vi "getPositionWithTime_32Bit.vi"(0 "connection ID":refnum<k5>, 1 "axis":i32, 5 "error":errorcluster) -> (14 "connection ID out":refnum<k5>, 15 "axis_out":i32, 16 "Monotonic_time_sec":i32, 17 "Monotonic_time_nsec":i32, 18 "position":dbl, 19 "error out":errorcluster)   [LabVIEW 2016, in "amc_api.lvlib"]
doc: "This function gets the current position of the positioner and provides time-information to the position."
uses:
  amc_api.lvlib
panel:
  out "jsonRespIn":string
  out "JSON-response":string="{\"jsonrpc\":\"2.0\",\"method\":\"\",\"params\":[5,1.245,true,\"name\"],\"id\":\"1\"}"
  out "JSON request":string
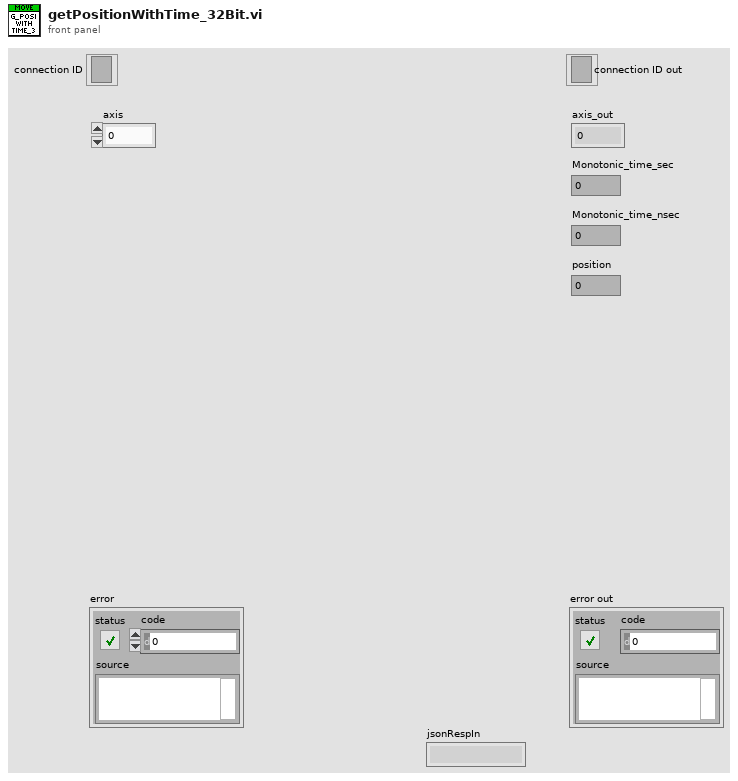
[diagram p1: front panel]
types:
  T1 = cluster{"jsonrpc":string, "method":string, "params":string[], "id":string, "api":i32, "pid":string}
  T2 = enum16{"Standard", "Buffered", "CRLF", "Immediate"}
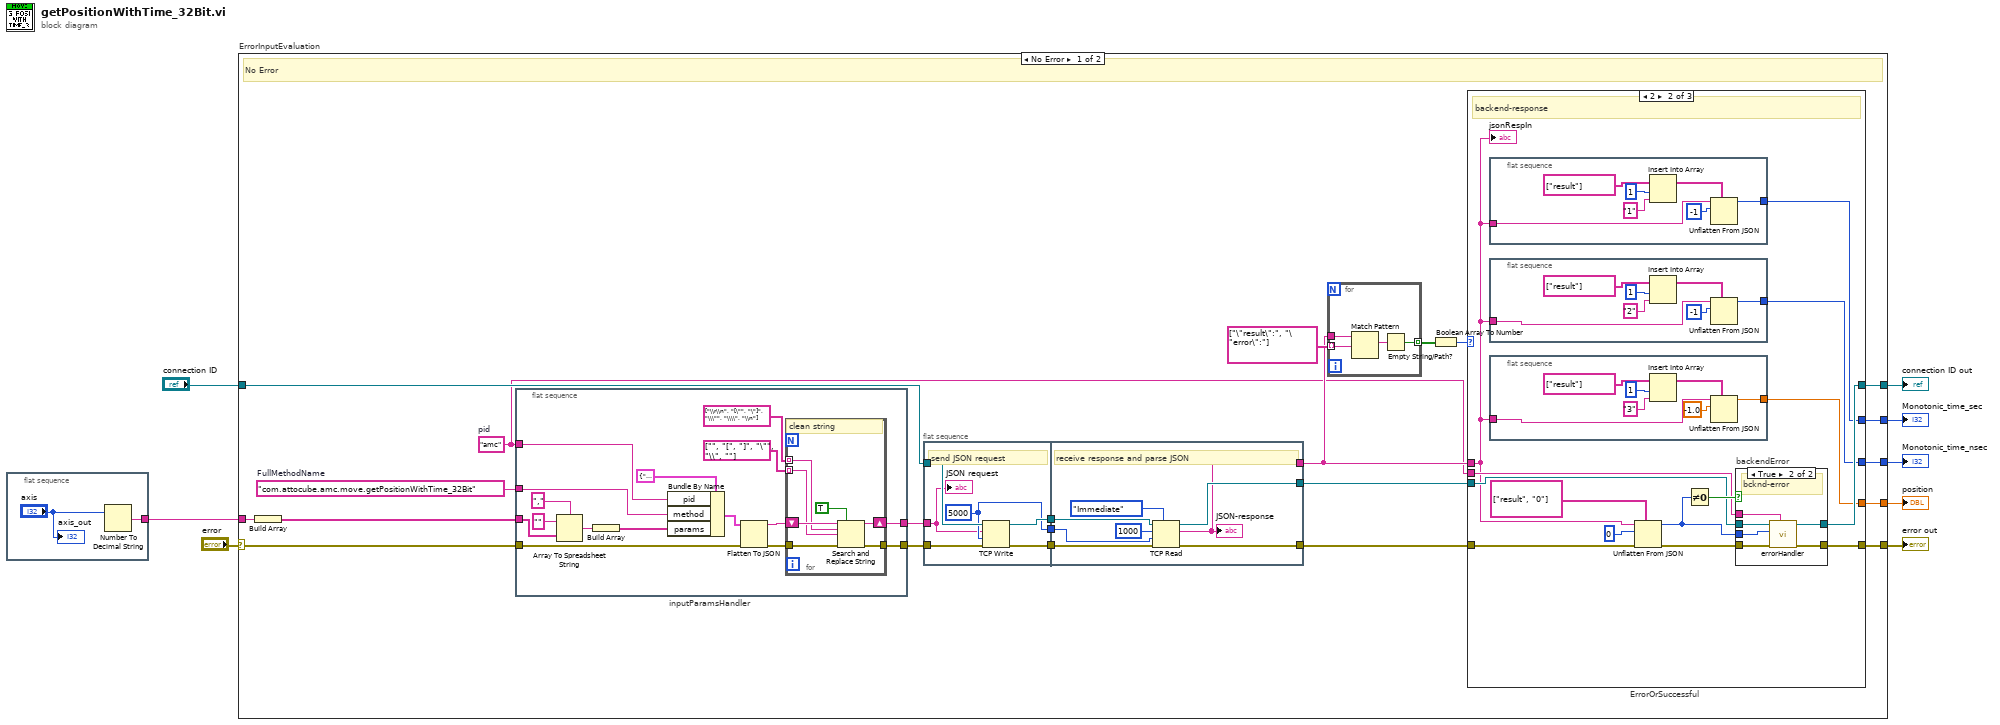
[diagram p0: block diagram]
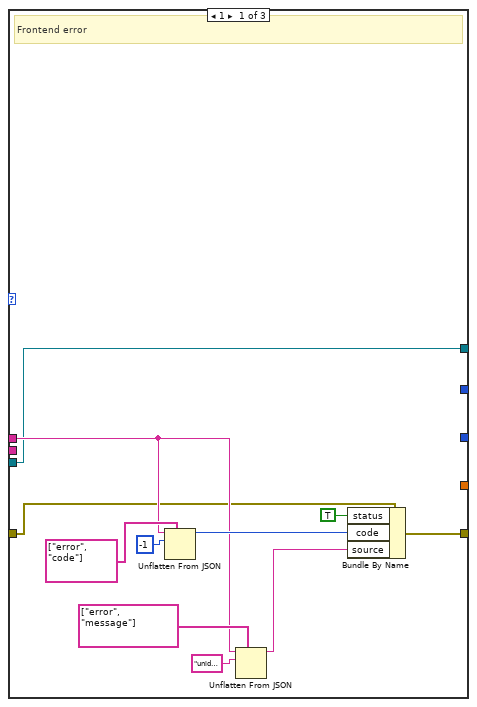
[diagram p2: hidden frame]
diagram:
  n1 = flat-sequence "in_axis" {
    tunnel: [w10] -> w4
    frame #0 {
      n2 = Number To Decimal String(number="axis") -> (decimal integer string=w10:string)  [unwired: 1 in]
      "axis_out" <- "axis"
    }
  }
  n3 = case "ErrorInputEvaluation" shown="No Error" "error" {
    selector: "error" -> [w25 w130]
    tunnel: "connection ID" -> [w29 w131]
    tunnel: [w16 w130] -> w7
    tunnel: [w17 w131] -> w6
    tunnel: w4 -> [w14 _]
    tunnel: [w13 _] -> w3
    tunnel: [w12 _] -> w2
    tunnel: [w11 _] -> w1
    frame No Error {
      w15 = "amc"  # pid
      w26 = "com.attocube.amc.move.getPositionWithTime_32Bit"  # FullMethodName
      # "No Error"
      n4 = Build Array ("ParametersArrayString")(w14) -> (w24:string[])
      n5 = flat-sequence "inputParamsHandler" {
        tunnel: [w94] -> w23
        tunnel: w24 -> [w100]
        tunnel: w25 -> [w99]
        tunnel: [w96] -> w22
        tunnel: w26 -> [w90]
        tunnel: w15 -> [w89]
        frame #0 {
          n6 = Array To Spreadsheet String(delimiter (Tab)=",", array=w100, 3:"" ("format string")) -> (spreadsheet string=w102:string)
          n7 = Build Array "Build Array"(w102) -> (w91:string[])
          n8 = Bundle By Name(cluster=T1 {"jsonrpc"="2.0", "method"="com.attocube.amc.res.setRESReadOutFreq", "params"=[], "id"="1", "api"=2, "pid"=""} ("Cluster"), "pid"=w89, "method"=w90, "params"=w91) -> (w101:T1)
          n9 = Flatten To JSON(anything=w101, error in (no error)=w99) -> (JSON string=w95:string, 11:w97:errorcluster)  [unwired: 1 in]
          n10 = for {
            tunnel: string[] ["\\r\\n", "[\"", "\"]", "\\\"", "\\\\", "\\n"] ("search string") -> [w108] mode=indexing
            tunnel: string[] ["", "[", "]", "\"", "\\", ""] ("replace string (\"\")") -> [w107] mode=indexing
            shift-right: [w110] -> w94
            shift-left: w95 -> [w109]
            tunnel: w97 -> [w106]
            tunnel: [w105] -> w96
            # "clean string"
            n11 = Search and Replace String(replace all?=TRUE ("replace all? (F)"), input string=w109, search string=w108, replace string=w107, error in=w106) -> (result string=w110:string, error out=w105:errorcluster)  [unwired: 3 in, 2 out]
          }
        }
      }
      n12 = flat-sequence {
        tunnel: w29 -> [w121]
        tunnel: [w119] -> w32
        tunnel: [w120] -> w31
        tunnel: w22 -> [w116]
        tunnel: [w118] -> w30
        tunnel: w23 -> [w117]
        tunnel: [w125] -> w21
        tunnel: w32 -> [w127]
        tunnel: w31 -> [w126]
        tunnel: [w123] -> w20
        tunnel: w30 -> [w124]
        tunnel: [w122] -> w19
        frame #0 {
          w118 = 5000 ("timeout ms (25000)")
          # "send JSON request"
          n13 = TCP Write(connection ID=w121, data in=w117, error in (no error)=w116, 9:w118) -> (connection ID out=w119:refnum<k5>, error out=w120:errorcluster)  [unwired: 1 out]
          "JSON request" <- w117
        }
        frame #1 {
          # "receive response and parse JSON"
          n14 = TCP Read(connection ID=w127, bytes to read=1000, error in (no error)=w126, 7:T2."Immediate" ("mode (standard)"), 9:w124) -> (connection ID out=w125:refnum<k5>, data out=w122:string, error out=w123:errorcluster)
          "JSON-response" <- w122
        }
      }
      n15 = for {
        tunnel: string[] ["\"result\":", "\"error\":"] ("path") -> [w114] mode=indexing
        tunnel: [w112] -> w27 mode=indexing
        tunnel: w19 -> [w115]
        n16 = Match Pattern(string=w115, regular expression=w114) -> (match substring=w113:string)  [unwired: 1 in, 3 out]
        n17 = Empty String/Path?(string/path=w113) -> (empty?=w112:bool)
      }
      n18 = Boolean Array To Number(Boolean array=w27) -> (number=w18:u32)
      n19 = case "ErrorOrSuccessful" shown="2" w18 {
        tunnel: w19 -> [w35 w49 _]
        tunnel: w21 -> [w33 w51 w88]
        tunnel: [w33 w50 w88] -> w17
        tunnel: [w36 w47 w87] -> w16
        tunnel: w20 -> [w34 w48 w87]
        tunnel: w15 -> [_ w52 _]
        tunnel: [_ w46 _] -> w13
        tunnel: [_ w45 _] -> w12
        tunnel: [_ w44 _] -> w11
        frame 1 {
          # "Frontend error"
          n20 = Unflatten From JSON(path=string[] ["error", "code"], JSON string=w35, type and defaults=-1) -> (value=w42:i32)  [unwired: 4 in, 1 out]
          n21 = Unflatten From JSON(path=string[] ["error", "message"], JSON string=w35, type and defaults="unidentified error") -> (value=w43:string)  [unwired: 4 in, 1 out]
          n22 = Bundle By Name(cluster=w34, "status"=TRUE, "code"=w42, "source"=w43) -> (w36:errorcluster)
        }
        frame 2 {
          # "backend-response"
          n23 = flat-sequence "out_integer" {
            tunnel: w49 -> [w74]
            tunnel: [w72] -> w46
            frame #0 {
              n24 = Insert Into Array(array=string[] ["result"] ("path"), index=1, new element="1" ("idx")) -> (w76:string[])
              n25 = Unflatten From JSON(path=w76, JSON string=w74, type and defaults=-1 ("index")) -> (value=w72:i32)  [unwired: 4 in, 1 out]
            }
          }
          n26 = flat-sequence "out_integer" {
            tunnel: w49 -> [w67]
            tunnel: [w65] -> w45
            frame #0 {
              n27 = Insert Into Array(array=string[] ["result"] ("path"), index=1, new element="2" ("idx")) -> (w69:string[])
              n28 = Unflatten From JSON(path=w69, JSON string=w67, type and defaults=-1 ("index")) -> (value=w65:i32)  [unwired: 4 in, 1 out]
            }
          }
          n29 = flat-sequence "out_double" {
            tunnel: [w58] -> w44
            tunnel: w49 -> [w60]
            frame #0 {
              n30 = Insert Into Array(array=string[] ["result"] ("path"), index=1, new element="3" ("idx")) -> (w62:string[])
              n31 = Unflatten From JSON(path=w62, JSON string=w60, type and defaults=-1.0 ("index")) -> (value=w58:dbl)  [unwired: 4 in, 1 out]
            }
          }
          n32 = Unflatten From JSON(path=string[] ["result", "0"], JSON string=w49, type and defaults=0, error in (no error)=w48) -> (value=w53:i32, error out=w55:errorcluster)  [unwired: 3 in]
          n33 = Not Equal To 0?(x=w53) -> (x != 0?=w54:bool)
          n34 = case "backendError" shown="True" w54 {
            tunnel: w53 -> [_ w86]
            tunnel: w55 -> [w80 w85]
            tunnel: [w79 w84] -> w50
            tunnel: [w80 w83] -> w47
            tunnel: w51 -> [w79 w82]
            tunnel: w52 -> [_ w81]
            frame False {
              # "successful"
            }
            frame True {
              # "bcknd-error"
              n35 = call "errorHandler.vi"("pid"=w81, "error in"=w85, "errNbr"=w86, "connection ID"=w82) -> ("error out 2"=w83:errorcluster, "connection ID out"=w84:refnum<k5>)  [unwired: 6 in]
            }
          }
          "jsonRespIn" <- w49
        }
        frame Default {
          # "NoResponse"
        }
      }
    }
    frame Error {
      # "Error"
    }
  }
  "error out" <- w7
  "connection ID out" <- w6
  "Monotonic_time_sec" <- w3
  "Monotonic_time_nsec" <- w2
  "position" <- w1
